vi "Get harmonics.vi"(7 "Initialize?":bool, 8 "error in (no error)":errorcluster, 10 "data":waveform(dbl)[](array[waveform]), 11 "Lock-in settings":T1={"Sine Frequency, Hz"=0.0, "Time constant, s"=0.12500000000000006, "Low-pass filter"=enum."No filtering", "Output representation"=enum."Real/Imaginary", "Phases, deg"=[], "Low-pass filter Order"=1, "Decimating factor"=1, "Samples to Read"=10000, "Post-filter decimation"=1, "Blocks to average"=1, "Trig delay, points"=0, "Harmonics per channel"=[], "Amplitude scale"=enum."RMS"} {"Time constant, s" format="%.1e"}) -> (0 "error out":errorcluster, 2 "Harmonics":cluster{waveform(dbl)[]}[](array[cluster]), 3 "Lock-in settings out":T1={"Sine Frequency, Hz"=0.0, "Time constant, s"=0.12500000000000006, "Low-pass filter"=enum."No filtering", "Output representation"=enum."Real/Imaginary", "Phases, deg"=[], "Low-pass filter Order"=1, "Decimating factor"=1, "Samples to Read"=10000, "Post-filter decimation"=1, "Blocks to average"=1, "Trig delay, points"=0, "Harmonics per channel"=[], "Amplitude scale"=enum."RMS"} {"Time constant, s" format="%.1e"})   [LabVIEW 2020]
uses:
  Lockin Settings.ctl
  Harmonics per channel.ctl
  <vilib>/measure/NI_MABase.lvlib
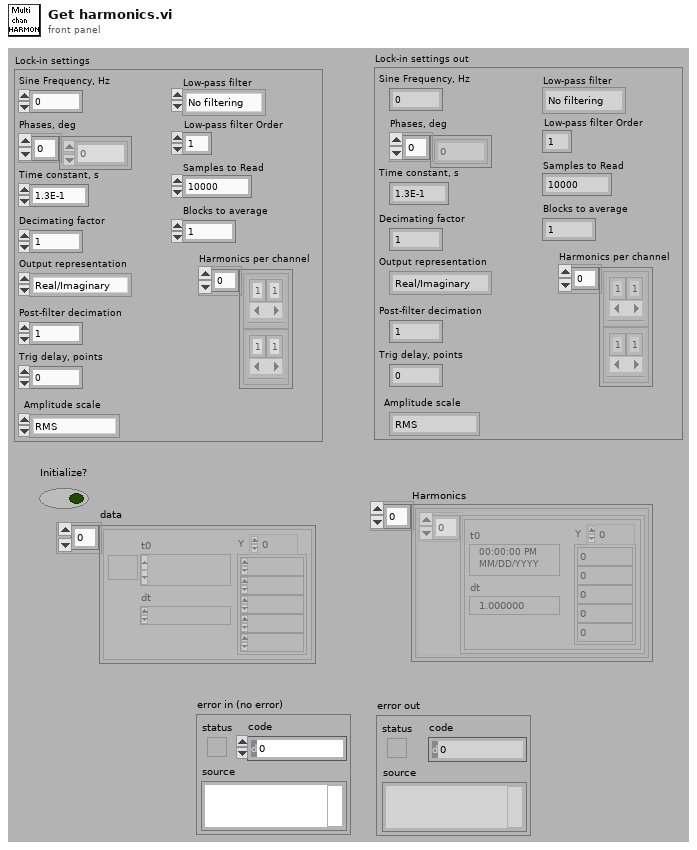
[diagram p1: front panel]
types:
  T1 = typedef "Lockin Settings.ctl" = cluster{"Sine Frequency, Hz":dbl, "Time constant, s":dbl, "Low-pass filter":enum16{"No filtering", "Butterworth", "Bessel"}, "Output representation":enum16{"Real/Imaginary", "Polar"}, "Phases, deg":dbl[], "Low-pass filter Order":i32, "Decimating factor":i32, "Samples to Read":i32, "Post-filter decimation":i32, "Blocks to average":i32, "Trig delay, points":i32, "Harmonics per channel":T2, "Amplitude scale":enum16{"Amplitude", "RMS", "Peak-to-Peak"}}
  T2 = typedef "Harmonics per channel.ctl" = cluster{"Harmonics":i32[]}[]
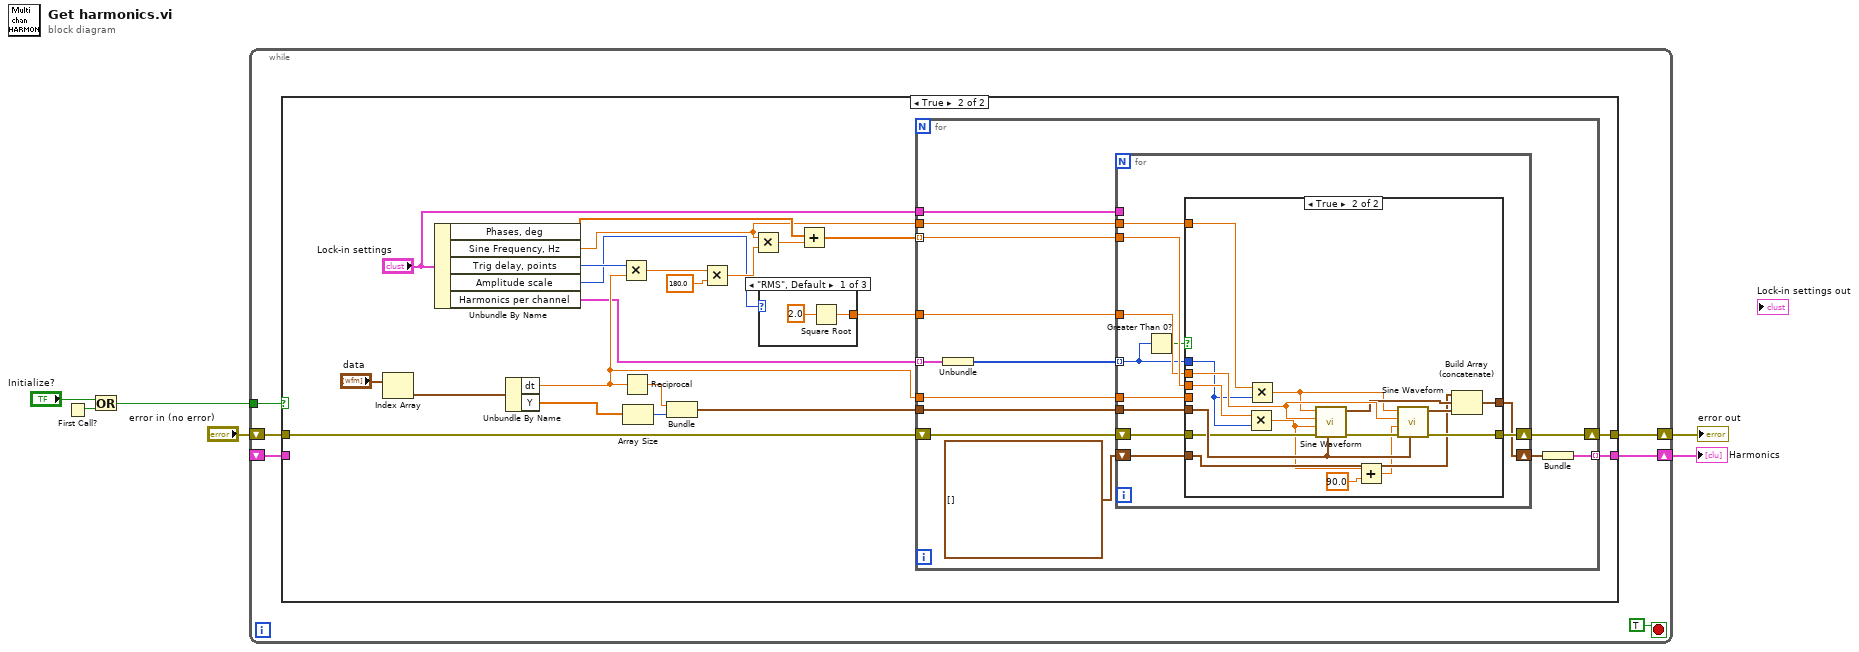
[diagram p0: block diagram]
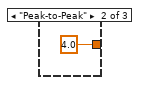
[diagram p3: hidden frame]
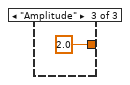
[diagram p4: hidden frame]
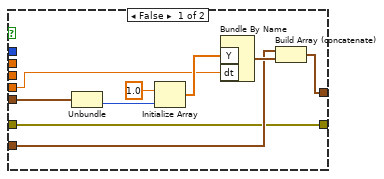
[diagram p5: hidden frame]
diagram:
  n1 = First Call?() -> (First Call?: T/F=w6:bool)
  n2 = Or(x="Initialize?", y=w6) -> (x .or. y?=w3:bool)
  n3 = while {
    tunnel: w3 -> [w10]
    shift-right: [w9] -> w2
    shift-left: "error in (no error)" -> [w12]
    shift-right: [w8] -> w1
    shift-left: _ -> [w7]
    stop <- TRUE stop-if-true
    n4 = case shown="True" w10 {
      tunnel: w12 -> [w13 w18]
      tunnel: [w13 w17] -> w9
      tunnel: [w14 w16] -> w8
      tunnel: w7 -> [w14 _]
      frame False {
      }
      frame True {
        n5 = Index Array(array="data") -> (element=w33:waveform(dbl))  [unwired: 1 in]
        n6 = Unbundle By Name("Lock-in settings") -> ("Phases, deg"=w29:dbl[], "Sine Frequency, Hz"=w20:dbl, "Trig delay, points"=w30:i32, "Amplitude scale"=w24:enum16{"Amplitude", "RMS", "Peak-to-Peak"}, "Harmonics per channel"=w15:T2)
        n7 = Unbundle By Name(w33) -> ("dt"=w19:dbl, "Y"=w35:dbl[])
        n8 = Multiply(x=w30, y=w19) -> (x*y=w26:dbl)
        n9 = Reciprocal(x=w19) -> (1/x=w36:dbl)
        n10 = Array Size(array=w35) -> (size(s)=w34:i32)
        n11 = Bundle(w36, w34) -> (w31:cluster{dbl, i32})  [unwired: 1 out]
        n12 = Multiply(x=w26, y=180.0) -> (x*y=w27:dbl)
        n13 = Multiply(x=w20, y=w27) -> (x*y=w28:dbl)
        n14 = case shown="\"RMS\", Default" w24 {
          tunnel: [w37 4.0 ("1/x") 2.0 ("1/x")] -> w21
          frame "RMS", Default {
            n15 = Square Root(x=2.0 ("1/x")) -> (sqrt(x)=w37:dbl)
          }
          frame "Peak-to-Peak" {
          }
          frame "Amplitude" {
          }
        }
        n16 = Add(x=w29, y=w28) -> (x+y=w22:dbl[])
        n17 = for {
          tunnel: w15 -> [w53] mode=indexing
          tunnel: "Lock-in settings" -> [w51]
          tunnel: w31 -> [w50]
          shift-right: [w48] -> w17
          shift-left: w18 -> [w49]
          tunnel: w22 -> [w47] mode=indexing
          tunnel: w21 -> [w46]
          tunnel: w20 -> [w44]
          tunnel: w19 -> [w43]
          tunnel: [w42] -> w16 mode=indexing
          n18 = Unbundle(w53) -> ("Harmonics"=w52:i32[])
          n19 = for {
            tunnel: w52 -> [w55] mode=indexing
            tunnel: w51 -> [_]
            tunnel: w50 -> [w64]
            shift-right: [w62] -> w48
            shift-left: w49 -> [w63]
            tunnel: w47 -> [w61]
            tunnel: w46 -> [w60]
            shift-right: [w58] -> w45
            shift-left: waveform(dbl)[] [] -> [w59]
            tunnel: w44 -> [w56]
            tunnel: w43 -> [w54]
            n20 = Greater Than 0?(x=w55) -> (x > 0?=w57:bool)
            n21 = case shown="True" w57 {
              tunnel: w64 -> [w73 w88]
              tunnel: w63 -> [w65 w87]
              tunnel: [w65 w86] -> w62
              tunnel: w61 -> [_ w85]
              tunnel: w60 -> [_ w84]
              tunnel: w59 -> [w66 w81]
              tunnel: [w67 w80] -> w58
              tunnel: w56 -> [_ w79]
              tunnel: w55 -> [_ w77]
              tunnel: w54 -> [w69 _]
              frame False {
                n22 = Unbundle(w73) -> (w72:i32)  [unwired: 1 out]
                n23 = Initialize Array(1.0 ("element"), w72) -> (w70:dbl[])
                n24 = Bundle By Name("Y"=w70, "dt"=w69) -> (w68:waveform(dbl))  [unwired: 1 in]
                n25 = Build Array (concatenate)(w66, w68) -> (w67:waveform(dbl)[])
              }
              frame True {
                n26 = Multiply(x=w85, y=w77) -> (x*y=w74:dbl)
                n27 = Multiply(x=w79, y=w77) -> (x*y=w78:dbl)
                n28 = call <vilib>:"Sine Waveform.vi"("sampling info"=w88, "error in (no error)"=w87, "phase"=w74, "amplitude"=w84, "frequency"=w78) -> ("error out"=w89:errorcluster, "signal out"=w83:waveform(dbl))  [unwired: 2 in, 3 out]
                n29 = Add(x=w74, y=90.0) -> (x+y=w75:dbl)
                n30 = call <vilib>:"Sine Waveform.vi"("sampling info"=w88, "error in (no error)"=w89, "phase"=w75, "amplitude"=w84, "frequency"=w78) -> ("error out"=w86:errorcluster, "signal out"=w82:waveform(dbl))  [unwired: 2 in, 3 out]
                n31 = Build Array (concatenate)(w81, w83, w82) -> (w80:waveform(dbl)[])
              }
            }
          }
          n32 = Bundle(w45) -> (w42:cluster{waveform(dbl)[]})  [unwired: 1 in]
        }
      }
    }
  }
  "error out" <- w2
  "Harmonics" <- w1
